vi "strassen_Kreuzungen.vi"(10 "Kreuzungen in":T1[](array[typedef]), 11 "Table Control":string[][](array[string])) -> (2 "Strassen":T3[](array[typedef]), 3 "Kreuzungen out":T1[](array[typedef]))   [LabVIEW 2019]
uses:
  Kreuzung.ctl
  Koordinate.ctl
  Strasse.ctl
  Verbindung.ctl
  Strassentyp.ctl
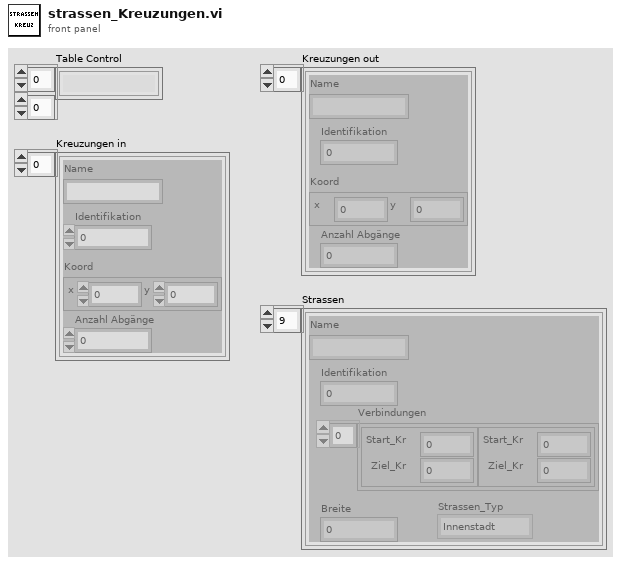
[diagram p1: front panel]
types:
  T1 = typedef "Kreuzung.ctl" = cluster{"Name":string, "Identifikation":u8, "Koord":T2, "Anzahl Abgänge":u8}
  T2 = typedef "Koordinate.ctl" = cluster{"x":dbl, "y":dbl}
  T3 = typedef "Strasse.ctl" = cluster{"Name":string, "Identifikation":u8, "Verbindungen":T4[], "Breite":u8, "Strassen_Typ":T5}
  T4 = typedef "Verbindung.ctl" = cluster{"Start_Kr":u16, "Ziel_Kr":u16}
  T5 = typedef "Strassentyp.ctl" = enum16{"Innenstadt", "Stadt", "Land"}
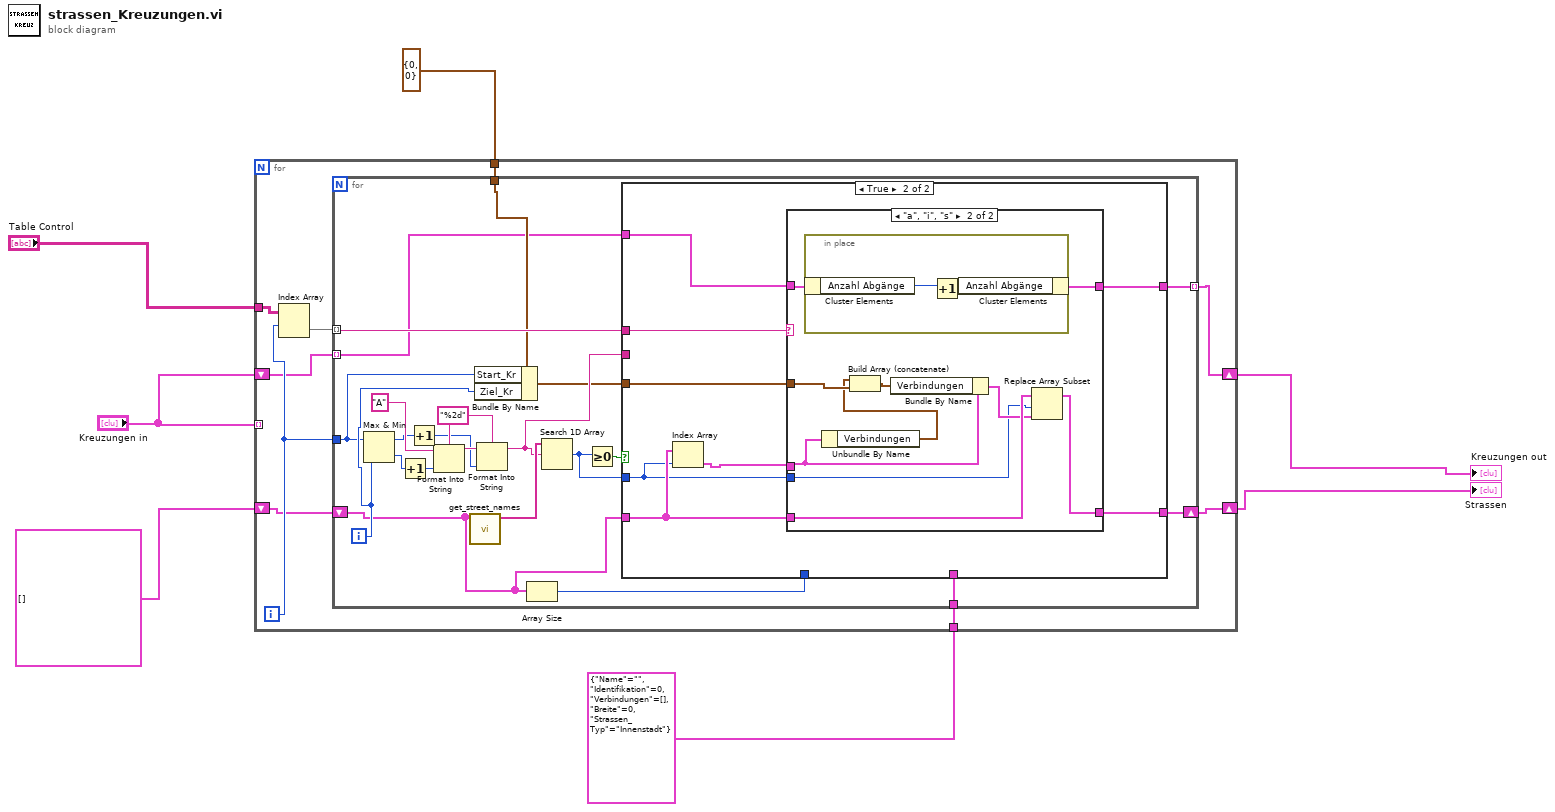
[diagram p0: block diagram]
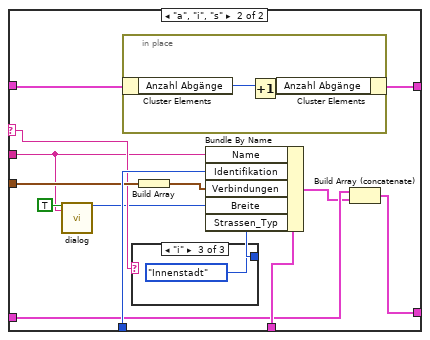
[diagram p3: hidden frame]
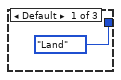
[diagram p4: hidden frame]
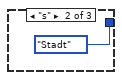
[diagram p5: hidden frame]
diagram:
  n1 = for {
    tunnel: "Kreuzungen in" -> [_] mode=indexing
    tunnel: "Table Control" -> [w16]
    shift-right: [w8] -> w7
    shift-left: "Kreuzungen in" -> [w9]
    shift-right: [w10] -> w6
    shift-left: T3[] [] ("Strassen") -> [w13]
    tunnel: T4 {"Start_Kr"=0, "Ziel_Kr"=0} ("Verbindung") -> [w12]
    tunnel: T3 {"Name"="", "Identifikation"=0, "Verbindungen"=[], "Breite"=0, "Strassen_Typ"=enum."Innenstadt"} ("Strasse") -> [w11]
    i -> [w14]
    n2 = Index Array(array=w16, index (row)=w14) -> (element=w15:string[])  [unwired: 1 in]
    n3 = for {
      tunnel: w15 -> [w38] mode=indexing
      tunnel: w14 -> [w30]
      shift-right: [w23] -> w10
      shift-left: w13 -> [w24]
      tunnel: w12 -> [w32]
      tunnel: w11 -> [w28]
      tunnel: w9 -> [w22] mode=indexing
      tunnel: [w21] -> w8 mode=indexing
      i -> [w31]
      w19 = "%2d" ("format string")
      n4 = Max & Min(x=w30, y=w31) -> (max(x,y)=w34:i32, min(x,y)=w37:i32)
      n5 = Increment(x=w37) -> (x+1=w17:i32)
      n6 = Increment(x=w34) -> (x+1=w18:i32)
      n7 = Format Into String(format string=w19, initial string="A", w17) -> (resulting string=w35:string)  [unwired: 1 in, 1 out]
      n8 = call "get_street_names.vi"("Strassen in"=w24) -> ("streets"=w33:string[])  [unwired: 10 in]
      n9 = Bundle By Name(cluster=w32, "Start_Kr"=w30, "Ziel_Kr"=w31) -> (w25:T4)
      n10 = Format Into String(format string=w19, initial string=w35, w18) -> (resulting string=w26:string)  [unwired: 1 in, 1 out]
      n11 = Array Size(array=w24) -> (size(s)=w27:i32)
      n12 = Search 1D Array(1D array=w33, element=w26) -> (index of element=w20:i32)  [unwired: 1 in]
      n13 = Greater Or Equal To 0?(x=w20) -> (x >= 0?=w29:bool)
      n14 = case shown="True" w29 {
        tunnel: w38 -> [w44 w75]
        tunnel: w28 -> [w47 _]
        tunnel: w27 -> [w46 _]
        tunnel: w26 -> [w39 _]
        tunnel: w25 -> [w45 w76]
        tunnel: w24 -> [w41 w71]
        tunnel: [w40 w72] -> w23
        tunnel: w22 -> [w43 w74]
        tunnel: [w42 w73] -> w21
        tunnel: w20 -> [_ w69]
        frame False {
          n15 = case shown="Default" w44 {
            selector: w44 -> [_ w53]
            tunnel: w47 -> [_ w63]
            tunnel: w46 -> [_ w62]
            tunnel: w39 -> [_ w51]
            tunnel: w45 -> [_ w61]
            tunnel: w43 -> [w49 w58]
            tunnel: [w49 w57] -> w42
            tunnel: w41 -> [w48 w56]
            tunnel: [w48 w54] -> w40
            frame Default {
            }
            frame "a", "i", "s" {
              n16 = call "dialog.vi"("Enable"=TRUE, "Strasse"=w51) -> ("Breite"=w50:u8)  [unwired: 17 in]
              n17 = in-place {
                n18 = in-place-cluster #1(w58) -> ("Anzahl Abgänge"=w68:u8)
                n19 = Increment(x=w68) -> (x+1=w67:u8)
                n20 = in-place-cluster #1("Anzahl Abgänge"=w67) -> (w57:T1)
              }
              n21 = case shown="\"i\"" w53 {
                tunnel: [Strassentyp."Land" ("Strassen_Typ") Strassentyp."Stadt" ("Strassen_Typ") Strassentyp."Innenstadt" ("Strassen_Typ")] -> w59
                frame Default {
                }
                frame "s" {
                }
                frame "i" {
                }
              }
              n22 = Build Array(w61) -> (w60:T4[])
              n23 = Bundle By Name(cluster=w63, "Name"=w51, "Identifikation"=w62, "Verbindungen"=w60, "Breite"=w50, "Strassen_Typ"=w59) -> (w55:T3)
              n24 = Build Array (concatenate)(w56, w55) -> (w54:T3[])
            }
          }
        }
        frame True {
          n25 = Index Array(array=w71, index=w69) -> (element=w70:T3)
          n26 = case shown="\"a\", \"i\", \"s\"" w75 {
            tunnel: w70 -> [_ w82]
            tunnel: w76 -> [_ w88]
            tunnel: w74 -> [w78 w86]
            tunnel: [w78 w85] -> w73
            tunnel: w71 -> [w77 w84]
            tunnel: [w77 w83] -> w72
            tunnel: w69 -> [_ w79]
            frame Default {
            }
            frame "a", "i", "s" {
              n27 = in-place {
                n28 = in-place-cluster #2(w86) -> ("Anzahl Abgänge"=w90:u8)
                n29 = Increment(x=w90) -> (x+1=w89:u8)
                n30 = in-place-cluster #2("Anzahl Abgänge"=w89) -> (w85:T1)
              }
              n31 = Unbundle By Name(w82) -> ("Verbindungen"=w81:T4[])
              n32 = Build Array (concatenate)(w81, w88) -> (w87:T4[])
              n33 = Bundle By Name(cluster=w82, "Verbindungen"=w87) -> (w80:T3)
              n34 = Replace Array Subset(array=w84, new element=w80, index=w79) -> (w83:T3[])
            }
          }
        }
      }
    }
  }
  "Kreuzungen out" <- w7
  "Strassen" <- w6
